vi "Drop n Messages.vi"(10 "n messages":i32, 11 "Sys Log in":refnum<class "System Log.lvclass">) -> (3 "Sys Log out":refnum<class "System Log.lvclass">)   [LabVIEW 2016, in "System Log.lvclass"]
uses:
  System Log.lvclass
  System Log.lvclass/System Log.ctl
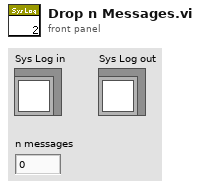
[diagram p1: front panel]
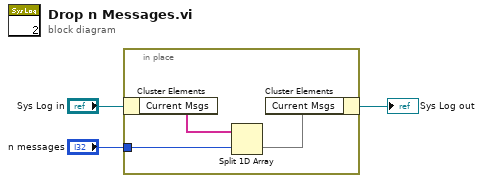
[diagram p0: block diagram]
diagram:
  n1 = in-place {
    in-place-border: "n messages" -> [w5]
    n2 = in-place-cluster #1("Sys Log in") -> ("Current Msgs"=w6:string[])
    n3 = Split 1D Array(array=w6, index=w5) -> (second subarray=w4:string[])  [unwired: 1 out]
    n4 = in-place-cluster #1("Current Msgs"=w4) -> (→"Sys Log out":refnum<class "System Log.lvclass">)
  }
